vi "worksheet set margins.vi"(6 "bottom":dbl, 7 "top":dbl, 8 "error in (no error)":errorcluster, 9 "right":dbl, 10 "left":dbl, 11 "worksheet":u32) -> (0 "error out":errorcluster)   [LabVIEW 2015, in "xlsxwriter.lvlib"]
doc: "void worksheet_set_margins(lxw_worksheet worksheet, double left, double right, double top, double bottom);"
uses:
  xlsxwriter.lvlib
  xlsxwriter.dll
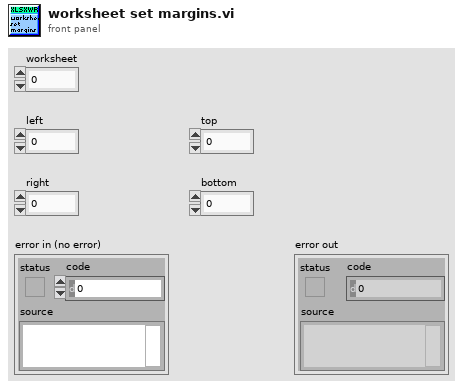
[diagram p1: front panel]
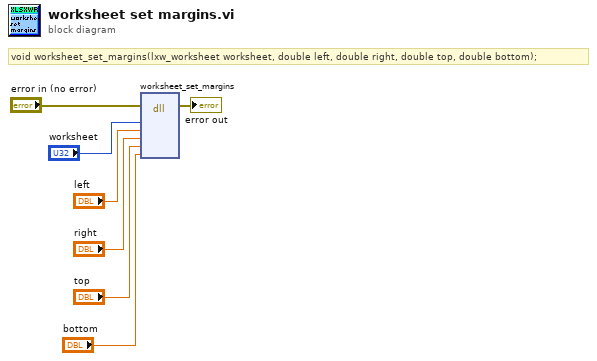
[diagram p0: block diagram]
diagram:
  # "void worksheet_set_margins(lxw_worksheet worksheet, double left, double right, double top, double bottom);"
  n1 = dll-call lib="C:/Users/WDAGUtilityAccount/Desktop/lv_vis_added_cell/xlsxwriter.*" fn="worksheet_set_margins"(error in="error in (no error)", "worksheet"="worksheet", "left"="left", "right"="right", "top"="top", "bottom"="bottom") -> (error out=→"error out":errorcluster)  [unwired: 8 in, 1 out]
